vi "Append Phrase.vi"(0 "PDF Report IN":T21(xcontrol), 2 "Text":string, 11 "error in (no error)":errorcluster, 12 "Font":T2={"Name"="", "Size"=-1.0, "Color"=0, "Style"={"Bold"=FALSE, "Italic"=FALSE, "Underline"=FALSE, "Strikeout"=FALSE}}, 14 "Line spacing":T1) -> (4 "PDF Report OUT":T21(xcontrol), 15 "error out":errorcluster)   [LabVIEW 2013]
doc: "Appends text to the PDF report. This text <B>can not</B> be aligned and indented. \n\nIf <B>Font</B> is not specified then the <B>Default font</B> will be use.\n\nThe data type you wire to the <B>Text</B> input determines the polymorphic instance to use.\n\n<B>FRANÇAIS</B>\nAjoute du texte au rapport. Ce texte ne peut être <B>aligné</B> et ne peut avoir un <B>renfoncement</B>.\n\nSi la police de caractères <B>Font</B> n'est pas spécifiée alors la <B>police de caractères par défaut</B> sera utilisée.\n\nLe type de données que vous connectez au terminal <B>Text</B> détermine l'instance polymorphique utilisée.\n\nDeveloped by Jean-Marc Simard\nCopyright © 2010, Exaprom Inc.\nAll rights reserved.\nLicense: BSD\n\nWith iTextSharp 4.1.6 (http://itextsharp.sourceforge.net)\nunder Mozilla Public License Version 1.1\n(http://www.mozilla.org/MPL/MPL-1.1.html)"
uses:
  Controls/Font cluster.ctl
  Controls/Font size.ctl
  Controls/Font color.ctl
  Controls/PDF Report Xcontrol/PDF Report.xctl
  Controls/Line spacing.ctl
  Controls/Texte alignement.ctl
  C:/Users/MaxCorp/Documents/GitHub/TopView/DLL/itextsharp.dll
  DLL/itextsharp.dll
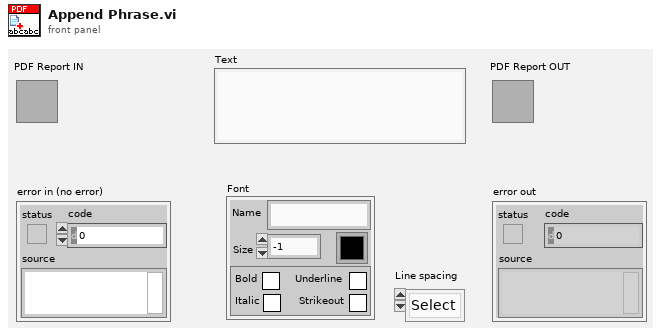
[diagram p1: front panel]
types:
  T1 = typedef "Line spacing.ctl" = enum16{"Select", "1.0", "1.5", "2.0"}
  T2 = typedef "Font cluster.ctl" = cluster{"Name":string, "Size":T3, "Color":T4, "Style":cluster{"Bold":bool, "Italic":bool, "Underline":bool, "Strikeout":bool}}
  T3 = typedef "Font size.ctl" = sgl
  T4 = typedef "Font color.ctl" = u32
  T5 = typedef "Unit.ctl" = enum16{"inch", "mm"}
  T6 = typedef "Paragraphe cluster.ctl" = cluster{" Aligment":T7, "Line spacing":T1}
  T7 = typedef "Texte alignement.ctl" = enum16{"Select", "CENTER", "JUSTIFY", "LEFT", "RIGHT"}
  T8 = typedef "Page dimensions.ctl" = cluster{"Start at page":i32, "Orientation":T9, "widht":sgl, "height":sgl, "Margin left":sgl, "Margin right":sgl, "Margin top":sgl, "Margin bottom":sgl}
  T9 = typedef "Page Orientation.ctl" = enum16{"Portrait", "Landscape"}
  T10 = typedef "Image or Table Caption.ctl" = cluster{"Caption":string, "Separator":string, "Position":enum16{"Above", "Below"}}
  T11 = typedef "Header Footer [ ].ctl" = T12[]
  T12 = typedef "Header Footer cluster.ctl" = cluster{"Start page":i32, "Type":T13, "Alignment":T14, "Vertical Alignement":T15, "Image (%)":sgl, "Page #":T16, "Text":string, "Path":string, "Font":T2, "Font refnum":refnum<k24>, "Line":cluster{"Line":T17, "Thickness (points)":sgl, "Colour":T4}}
  T13 = typedef "Header Footer Type.ctl" = enum16{"Select", "Text", "Text + hyperlink", "Page number", "Image", "Image + hyperlink"}
  T14 = typedef "Header footer horiz alignment.ctl" = enum16{"Left", "Center", "Right"}
  T15 = typedef "Cell Vertical alignment.ctl" = enum16{"TOP", "MIDDLE", "BOTTOM"}
  T16 = typedef "Page number.ctl" = cluster{"Text 1":string, "Text 2":string, "Text 3":string}
  T17 = typedef "Header Footer Line.ctl" = enum16{"No line", "Horizontal line"}
  T18 = typedef "Watermark cluster2.ctl" = cluster{"Show? (F)":bool, "Type":enum16{"Image", "Text"}, "Opacity (%)":sgl, "Rotate(°)":sgl, "Position":cluster{"Position":T19, "X":sgl, "Y":sgl}, "Image path":path, "Scaled(%)":sgl, "Image refnum":refnum<k24>, "Text":string, "Font":cluster{"Name":string, "Size":T3, "Color":T4}, "Font refnum":refnum<k24>, "Alignment":T14, "Automatic":bool}
  T19 = typedef "Watermark Position.ctl" = enum16{"Absolute", "Center (page)", "Center (text section)"}
  T20 = typedef "System Fonts.ctl" = cluster{"Font name [ ]":string[], "Font and file names [ ]":cluster{"Font name":string, "File name":string}[]}
  T21 = cluster{"Document":refnum<k24>, "Writer":refnum<k24>, "Default Font":refnum<k24>, "Default Font cluster":T2, "Path":path, "Unit (default = mm)":T5, "Paragraphe cluster":T6, "Pages dimensions [ ]":T8[], "Captions":cluster{"Image":T10, "Image counter":u16, "Table":T10, "Table counter":u16, "Font":T2}, "Header":T11, "Footer":T11, "Watermark ":T18, "Actual VI name":string, "System Fonts":T20}
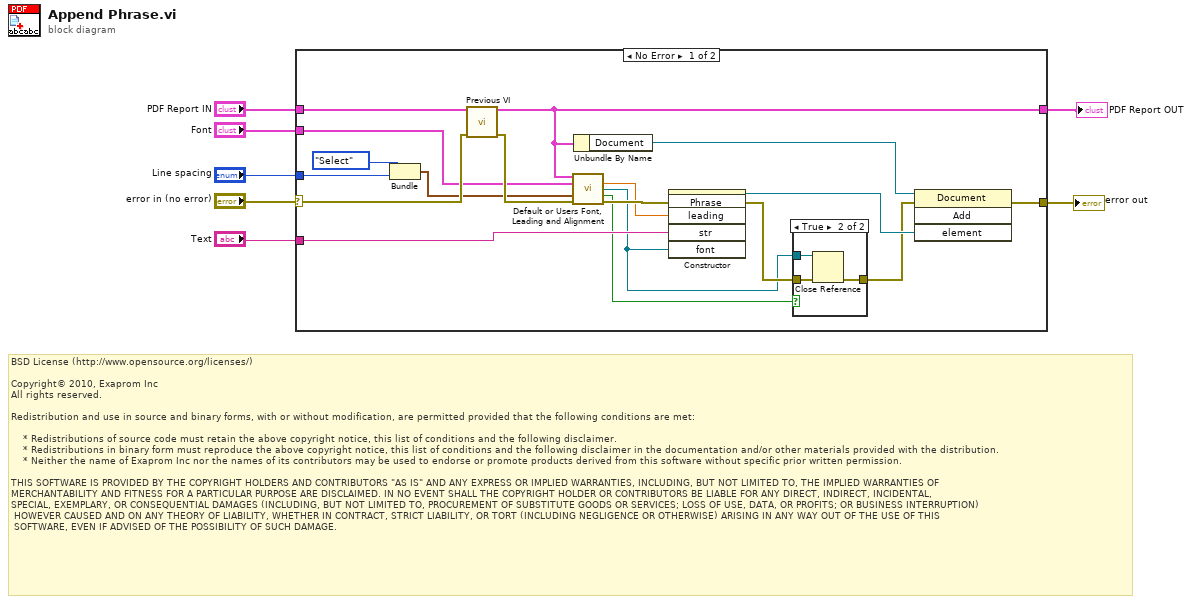
[diagram p0: block diagram]
diagram:
  # "BSD License (http://www.opensource.org/licenses/)\n\nCopyright© 2010, Exaprom Inc\nAll rights reserved.\n\nRedistribution and use in source and binary forms, with or without modification, are permitted provided that the following conditions are met:\n\n    * Redistributions of source code must retain the above copyright notice, this list of conditions and the following disclaimer.\n    * Redistributions in binary form must reproduce the above copyright notice, this list of conditions and the following disclaimer in the documentation and/or other materials provided with the distribution.\n    * Neither the name of Exaprom Inc nor the names of its contributors may be used to endorse or promote products derived from this software without specific prior written permission.\n\nTHIS SOFTWARE IS PROVIDED BY THE COPYRIGHT HOLDERS AND CONTRIBUTORS \"AS IS\" AND ANY EXPRESS OR IMPLIED WARRANTIES, INCLUDING, BUT NOT LIMITED TO, THE IMPLIED WARRANTIES OF \nMERCHANTABILITY AND FITNESS FOR A PARTICULAR PURPOSE ARE DISCLAIMED. IN NO EVENT SHALL THE COPYRIGHT HOLDER OR CONTRIBUTORS BE LIABLE FOR ANY DIRECT, INDIRECT, INCIDENTAL,\nSPECIAL, EXEMPLARY, OR CONSEQUENTIAL DAMAGES (INCLUDING, BUT NOT LIMITED TO, PROCUREMENT OF SUBSTITUTE GOODS OR SERVICES; LOSS OF USE, DATA, OR PROFITS; OR BUSINESS INTERRUPTION)\n HOWEVER CAUSED AND ON ANY THEORY OF LIABILITY, WHETHER IN CONTRACT, STRICT LIABILITY, OR TORT (INCLUDING NEGLIGENCE OR OTHERWISE) ARISING IN ANY WAY OUT OF THE USE OF THIS\n SOFTWARE, EVEN IF ADVISED OF THE POSSIBILITY OF SUCH DAMAGE."
  n1 = case shown="No Error" "error in (no error)" {
    selector: "error in (no error)" -> [w25 w31]
    tunnel: "Font" -> [w20 _]
    tunnel: [w8 w30] -> w1
    tunnel: [w23 w31] -> w2
    tunnel: "PDF Report IN" -> [w21 w30]
    tunnel: "Line spacing" -> [w18 _]
    tunnel: "Text" -> [w15 _]
    frame No Error {
      n2 = Bundle("Aligment"=Texte_alignement."Select", "Line spacing"=w18) -> (w17:cluster{"Aligment":T7, "Line spacing":T1})  [unwired: 1 out]
      n3 = call "Previous VI.vi"("PDF Report IN"=w21, "error in (no error)"=w25) -> ("PDF Report OUT"=w8:T21, "error out"=w24:errorcluster)  [unwired: 12 out]
      n4 = call "Default or Users Font, Leading and Alignment.vi"("PDF Report"=w8, "Font"=w20, "Paragraphe cluster"=w17, "error in (no error)"=w24) -> ("Leading"=w16:T3, "Font Ref"=w9:refnum<k24>, "Close Font Ref"=w10:bool, "error out"=w22:errorcluster)  [unwired: 8 out]
      n5 = Unbundle By Name(w8) -> ("Document"=w19:refnum<k24>)
      n6 = constructor class="Phrase"(error in=w22, "leading"=w16, "str"=w15, "font"=w9) -> (reference out=w14:refnum<k24>, error out=w12:errorcluster)  [unwired: 2 in, 4 out]
      n7 = case shown="True" w10 {
        tunnel: w9 -> [_ w29]
        tunnel: w12 -> [w26 w28]
        tunnel: [w26 w27] -> w11
        frame False {
        }
        frame True {
          n8 = Close Reference(reference=w29, error in (no error)=w28) -> (error out=w27:errorcluster)
        }
      }
      n9 = invoke class="Document" method="Add"(reference=w19, error in=w11, "element"=w14) -> (error out=w23:errorcluster)  [unwired: 1 in, 3 out]
    }
    frame Error {
    }
  }
  "PDF Report OUT" <- w1
  "error out" <- w2
